vi "NXT ReadData.vi"(3 "error in (no error)":errorcluster) -> (0 "error out":errorcluster, 1 "Valid String?":bool, 2 "Data Out":u8[](array[numeric]))   [LabVIEW 2012]
doc: "This is an NXT vi. I reads data from the NXTBEE and output the result as an array of bytes. It also outputs a valid sting flag."
uses:
  <vilib>/NXT/NXT Controls/NXTSyscallRefnum.ctl
  <resource>/objmgr/NXTInputOutput.rc
panel:
  in  "Sys Call Refnum":T1
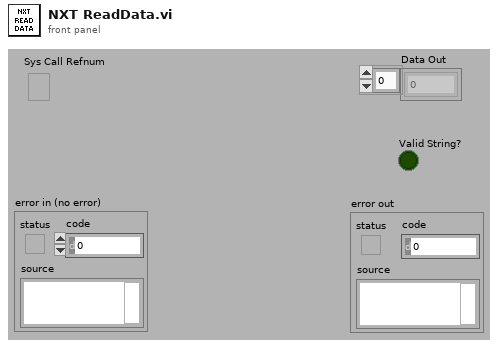
[diagram p1: front panel]
types:
  T1 = typedef "NXTSyscallRefnum.ctl" = refnum<k21>
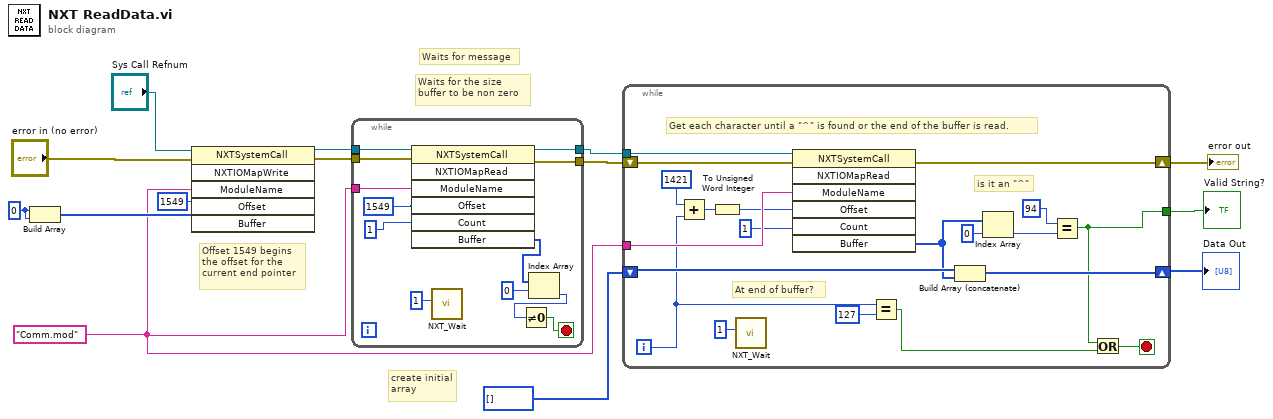
[diagram p0: block diagram]
diagram:
  w3 = u8 0 ("element")
  w4 = "Comm.mod" ("ModuleName")
  # "create initial\narray"
  # "Waits for message"
  # "Waits for the size\nbuffer to be non zero"
  # "Offset 1549 begins\nthe offset for the\ncurrent end pointer"
  n1 = Build Array(w3, w3) -> (w11:u8[])
  n2 = invoke class="NXTSystemCall" method="NXTIOMapWrite"(reference="Sys Call Refnum", error in="error in (no error)", "ModuleName"=w4, "Offset"=u16 1549, "Buffer"=w11) -> (reference out=w2:T1, error out=w5:errorcluster)  [unwired: 1 in, 4 out]
  n3 = while {
    tunnel: [w22] -> w7
    tunnel: [w21] -> w6
    tunnel: w2 -> [w20]
    tunnel: w5 -> [w19]
    tunnel: w4 -> [w18]
    stop <- w17 stop-if-true
    n4 = invoke class="NXTSystemCall" method="NXTIOMapRead"(reference=w20, error in=w19, "ModuleName"=w18, "Offset"=u16 1549, "Count"=u16 1) -> (reference out=w22:T1, error out=w21:errorcluster, "Buffer"=w25:u8[])  [unwired: 2 in, 4 out]
    n5 = call <vilib>:"NXT_Wait.vi"("Wait (ms)"=u32 1) -> ()  [unwired: 9 in, 2 out]
    n6 = Index Array(array=w25, index=0) -> (element=w16:u8)
    n7 = Not Equal To 0?(x=w16) -> (x != 0?=w17:bool)
  }
  n8 = while {
    tunnel: w4 -> [w44]
    tunnel: w7 -> [w41]
    shift-right: [w46] -> w12
    shift-left: w6 -> [w40]
    shift-right: [w42] -> w8
    shift-left: u8[] [] -> [w37]
    tunnel: [w28] -> w1
    i -> [w36]
    stop <- w30 stop-if-true
    # "At end of buffer?"
    # "Get each character until a \"^\" is found or the end of the buffer is read."
    # "is it an \"^\""
    n9 = Add(x=1421 ("Offset"), y=w36) -> (x+y=w39:i32)
    n10 = To Unsigned Word Integer(number=w39) -> (unsigned 16bit integer=w38:u16)
    n11 = call <vilib>:"NXT_Wait.vi"("Wait (ms)"=u32 1) -> ()  [unwired: 9 in, 2 out]
    n12 = invoke class="NXTSystemCall" method="NXTIOMapRead"(reference=w41, error in=w40, "ModuleName"=w44, "Offset"=w38, "Count"=u16 1) -> (error out=w46:errorcluster, "Buffer"=w34:u8[])  [unwired: 2 in, 5 out]
    n13 = Equal?(x=w36, y=127) -> (x = y?=w29:bool)
    n14 = Build Array (concatenate)(w37, w34) -> (w42:u8[])
    n15 = Index Array(array=w34, index=0) -> (element=w32:u8)
    n16 = Equal?(x=u8 94, y=w32) -> (x = y?=w28:bool)
    n17 = Or(x=w28, y=w29) -> (x .or. y?=w30:bool)
  }
  "error out" <- w12
  "Data Out" <- w8
  "Valid String?" <- w1
